vi "Update Click Zones.vi"(7 "pixels per unit":dbl, 8 "error in (no error)":errorcluster, 9 "picture size (pixels)":T1={"Width"=500, "Height"=500}, 10 "click zones group in":T3, 11 "steering frame in":refnum<class "NI_Robotics_Steering Frame.lvclass">) -> (0 "error out":errorcluster, 2 "click zones group out":T3, 3 "steering frame out":refnum<class "NI_Robotics_Steering Frame.lvclass">)   [LabVIEW 2017, in "NI_Robotics_Configure Steering Frame.lvlib"]
uses:
  <vilib>/robotics/Dialog/Configure Steering Frame/NI_Robotics_Configure Steering Frame.lvlib
  <vilib>/robotics/Dialog/Configure Steering Frame/Click Zone.ctl
  <vilib>/Utility/miscctls.llb/LVBoundsTypeDef.ctl
  <vilib>/robotics/Steering/Steering Frame/NI_Robotics_Steering Frame.lvclass
  <vilib>/robotics/Steering/Steering Frame/NI_Robotics_Steering Frame.lvclass/NI_Robotics_Steering Frame.ctl
  <vilib>/robotics/Steering/Wheel/NI_Robotics_Wheel.lvclass
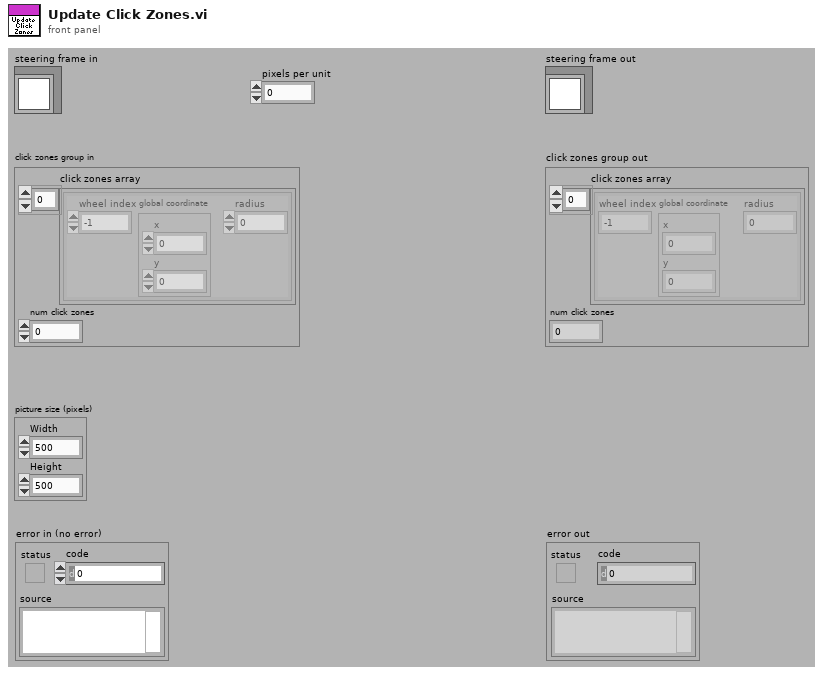
[diagram p1: front panel]
types:
  T1 = typedef "LVBoundsTypeDef.ctl" = cluster{"Width":u32, "Height":u32}
  T2 = typedef "NI_Robotics_Configure Steering Frame.lvlib/Click Zone.ctl" = cluster{"wheel index":i32, "global coordinate":cluster{"x":dbl, "y":dbl}, "radius":dbl}
  T3 = cluster{"click zones array":T2[], "num click zones":i32}
  T4 = cluster{"elements":T2[], "number of elements":i32}
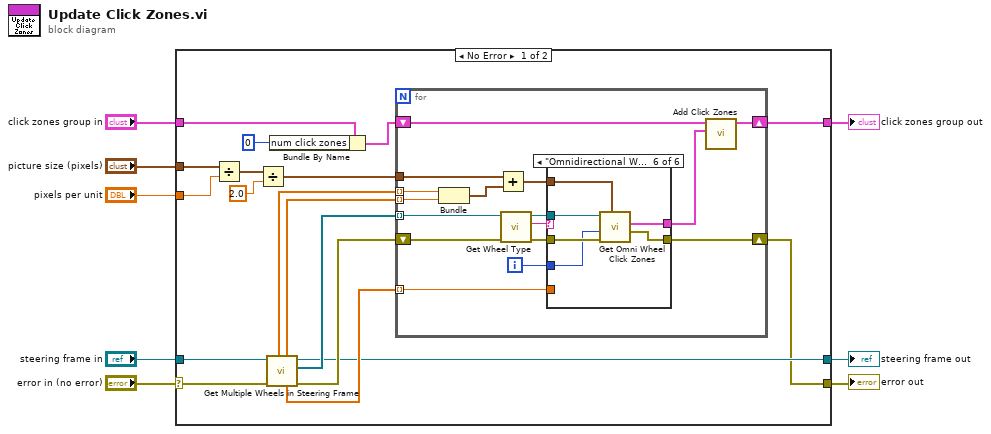
[diagram p0: block diagram]
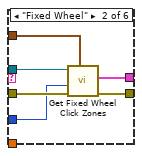
[diagram p3: hidden frame]
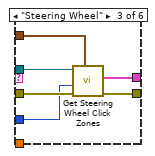
[diagram p4: hidden frame]
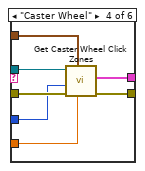
[diagram p5: hidden frame]
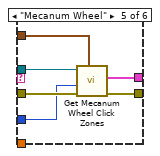
[diagram p6: hidden frame]
diagram:
  n1 = case shown="No Error" "error in (no error)" {
    selector: "error in (no error)" -> [w21 w77]
    tunnel: [w9 w77] -> w7
    tunnel: "click zones group in" -> [w20 w76]
    tunnel: [w17 w76] -> w5
    tunnel: "steering frame in" -> [w22 w75]
    tunnel: [w10 w75] -> w3
    tunnel: "picture size (pixels)" -> [w24 _]
    tunnel: "pixels per unit" -> [w23 _]
    frame No Error {
      n2 = Divide(x=w24, y=w23) -> (x/y=w26:cluster{"Width":dbl, "Height":dbl})
      n3 = Divide(x=w26, y=2.0) -> (x/y=w16:cluster{"Width":dbl, "Height":dbl})
      n4 = call <vilib>:"Get Multiple Wheels in Steering Frame.vi"("error in (no error)"=w21, "steering frame in"=w22) -> ("error out"=w12:errorcluster, "wheels"=w13:refnum<class "NI_Robotics_Wheel.lvclass">[], "steering frame out"=w10:refnum<class "NI_Robotics_Steering Frame.lvclass">, "frame angles (rad)"=w11:dbl[], "y positions"=w14:dbl[], "x positions"=w15:dbl[])  [unwired: 3 in, 1 out]
      n5 = Bundle By Name(cluster=w20, "num click zones"=0) -> (w18:T3)
      n6 = for {
        shift-right: [w28] -> w17
        shift-left: w18 -> [w29]
        tunnel: w16 -> [w37]
        tunnel: w15 -> [w36] mode=indexing
        tunnel: w14 -> [w35] mode=indexing
        tunnel: w13 -> [w34] mode=indexing
        shift-right: [w32] -> w9
        shift-left: w12 -> [w33]
        tunnel: w11 -> [w31] mode=indexing
        i -> [w30]
        n7 = Bundle("x position"=w36, "y position"=w35) -> (w41:cluster{"x position":dbl, "y position":dbl})  [unwired: 1 in]
        n8 = Add(x=w37, y=w41) -> (x+y=w42:cluster{dbl, dbl})
        n9 = call-dynamic "Get Wheel Type.vi"("error in (no error)"=w33, "wheel in"=w34) -> ("error out"=w39:errorcluster, "wheel type"=w38:string, "wheel out"=w40:refnum<class "NI_Robotics_Wheel.lvclass">)  [unwired: 7 in]
        n10 = case shown="\"Omnidirectional Wheel\"" w38 {
          tunnel: w39 -> [w43 w48 w54 w62 w67 w74]
          tunnel: w40 -> [_ w49 w55 w60 w68 w73]
          tunnel: [w43 w47 w53 w61 w66 w70] -> w32
          tunnel: w42 -> [_ w46 w51 w59 w64 w71]
          tunnel: w30 -> [_ w45 w52 w58 w65 w72]
          tunnel: w31 -> [_ _ _ w57 _ _]
          tunnel: [_ w44 w50 w56 w63 w69] -> w27
          frame "Wheel", Default {
          }
          frame "Fixed Wheel" {
            n11 = call <vilib>:"Get Fixed Wheel Click Zones.vi"("global wheel position"=w46, "error in (no error)"=w48, "wheel index"=w45, "wheel in"=w49) -> ("error out"=w47:errorcluster, "click zones"=w44:T2[])  [unwired: 5 in, 1 out]
          }
          frame "Steering Wheel" {
            n12 = call <vilib>:"Get Steering Wheel Click Zones.vi"("global wheel position"=w51, "error in (no error)"=w54, "wheel index"=w52, "wheel in"=w55) -> ("error out"=w53:errorcluster, "click zones"=w50:T2[])  [unwired: 5 in, 1 out]
          }
          frame "Caster Wheel" {
            n13 = call <vilib>:"Get Caster Wheel Click Zones.vi"("wheel frame angle (rad)"=w57, "global wheel position"=w59, "error in (no error)"=w62, "wheel index"=w58, "wheel in"=w60) -> ("error out"=w61:errorcluster, "click zones"=w56:T2[])  [unwired: 4 in, 1 out]
          }
          frame "Mecanum Wheel" {
            n14 = call <vilib>:"Get Mecanum Wheel Click Zones.vi"("global wheel position"=w64, "error in (no error)"=w67, "wheel index"=w65, "wheel in"=w68) -> ("error out"=w66:errorcluster, "click zones"=w63:T2[])  [unwired: 5 in, 1 out]
          }
          frame "Omnidirectional Wheel" {
            n15 = call <vilib>:"Get Omni Wheel Click Zones.vi"("global wheel position"=w71, "error in (no error)"=w74, "wheel index"=w72, "wheel in"=w73) -> ("error out"=w70:errorcluster, "click zones"=w69:T2[])  [unwired: 5 in, 1 out]
          }
        }
        n16 = call <vilib>:"Add Click Zones.vi"("click zones to add"=w27, "array in"=w29) -> ("array out"=w28:T4)  [unwired: 9 in]
      }
    }
    frame Error {
    }
  }
  "steering frame out" <- w3
  "error out" <- w7
  "click zones group out" <- w5
